vi "Get All Performance Channels from Section.vi"(8 "error in (no error)":errorcluster, 10 "Section Name":string, 11 "Item Ref in":T1 format="%.0x") -> (0 "error out":errorcluster, 2 "performance channels refs":T1[](array[typedef]) format="%.0x", 3 "Item Ref out":T1 format="%.0x")   [LabVIEW 2017, in "DSF Shared.lvlib"]
uses:
  DSF Shared.lvlib
  <vilib>/NI Veristand/Custom Device API/Custom Device Item Ref.ctl
  <vilib>/NI Veristand/Custom Device API/Custom Device API.lvlib
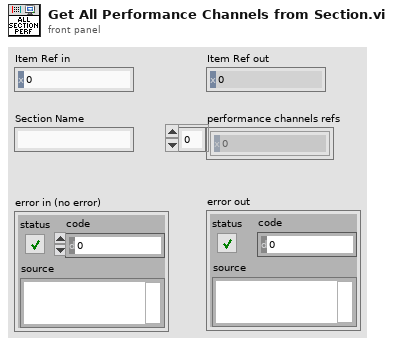
[diagram p1: front panel]
types:
  T1 = typedef "Custom Device API.lvlib/Custom Device Item Ref.ctl" = u64
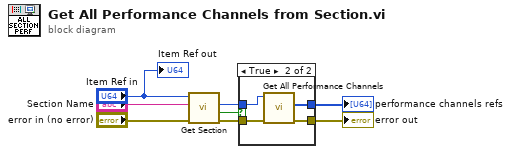
[diagram p0: block diagram]
diagram:
  n1 = call "Get Section.vi"("error in (no error)"="error in (no error)", "Section Name"="Section Name", "Item Ref in"="Item Ref in") -> ("error out"=w8:errorcluster, "found"=w7:bool, "Section ref"=w6:T1)  [unwired: 5 in, 1 out]
  n2 = case shown="True" w7 {
    tunnel: w8 -> [w9 w13]
    tunnel: w6 -> [_ w12]
    tunnel: [_ w11] -> w2
    tunnel: [w9 w10] -> w3
    frame False {
    }
    frame True {
      n3 = call "Get All Performance Channels.vi"("error in (no error)"=w13, "Item Ref in"=w12) -> ("error out"=w10:errorcluster, "Channels refs"=w11:T1[])  [unwired: 7 in, 1 out]
    }
  }
  "error out" <- w3
  "performance channels refs" <- w2
  "Item Ref out" <- "Item Ref in"
